vi "SL2_AD_DLL_Phoibos_SetDeviceState.vi"(4 "pHandle_in":u32, 5 "error in":errorcluster, 6 "state":T2 items=["Off"=-1, "Standby"=0, "On"=1], 7 "dev_type":T1, 8 "dll_path":path) -> (0 "error out":errorcluster, 3 "path out":path)   [LabVIEW 2020]
uses:
  DEFINITIONS/DEF_dev_state.ctl
  DEFINITIONS/DEF_dev_type.ctl
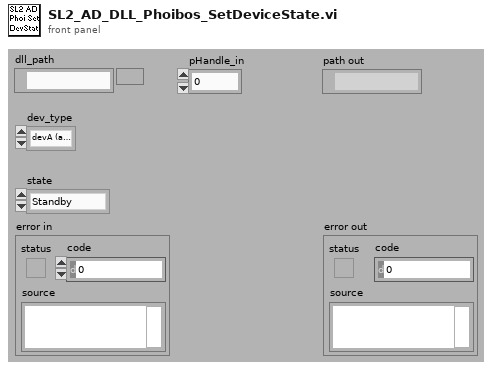
[diagram p1: front panel]
types:
  T1 = typedef "DEF_dev_type.ctl" = enum32{"devA (analyzer)", "devD (detector)"}
  T2 = typedef "DEF_dev_state.ctl" = i32
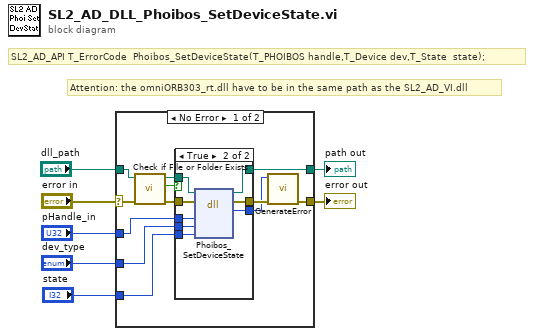
[diagram p0: block diagram]
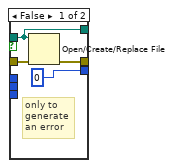
[diagram p2: hidden frame]
diagram:
  # "SL2_AD_API T_ErrorCode  Phoibos_SetDeviceState(T_PHOIBOS handle,T_Device dev,T_State  state);"
  # "Attention: the omniORB303_rt.dll have to be in the same path as the SL2_AD_VI.dll"
  n1 = case shown="No Error" "error in" {
    selector: "error in" -> [w16 w33]
    tunnel: "state" -> [w19 _]
    tunnel: "dev_type" -> [w18 _]
    tunnel: [w12 w33] -> w5
    tunnel: [w17 w32] -> w4
    tunnel: "dll_path" -> [w15 w32]
    tunnel: "pHandle_in" -> [w14 _]
    frame No Error {
      n2 = call <vilib>:"Check if File or Folder Exists.vi"("error in (no error)"=w16, "path"=w15) -> ("error out"=w10:errorcluster, "file or folder exists?"=w8:bool, "dup path"=w9:path)  [unwired: 7 in]
      n3 = case shown="True" w8 {
        tunnel: w19 -> [_ w29]
        tunnel: w18 -> [_ w30]
        tunnel: [w23 w26] -> w13
        tunnel: [w21 w24] -> w17
        tunnel: [u32 0 ("error_code") w28] -> w11
        tunnel: w10 -> [w22 w31]
        tunnel: w9 -> [w21 w25]
        tunnel: w14 -> [_ w27]
        frame False {
          # "only to generate an error"
          n4 = Open/Create/Replace File(file path (use dialog)=w21, error in=w22) -> (error out=w23:errorcluster)  [unwired: 4 in, 2 out]
        }
        frame True {
          n5 = dll-call lib="C:/Programme/SPECS/SpecsLab2/programming/LabView7.1/SL2_AD_VI.dll" fn="Phoibos_SetDeviceState"(path in=w25, error in=w31, "pHandle"=w27, "dev"=w30, "state"=w29) -> (path out=w24:path, error out=w26:errorcluster, "error_code"=w28:u32)  [unwired: 4 in]
        }
      }
      n6 = call "GenerateError.vi"("error in"=w13, "error_code"=w11) -> ("error out"=w12:errorcluster)  [unwired: 9 in]
    }
    frame Error {
    }
  }
  "error out" <- w5
  "path out" <- w4
